vi "RT_Angular Aceleration in DLR Navigation Reference System(SubVI).vi"(0 "Mco (Nm)":dbl[](array[numeric]), 1 "MFE (Nm)":dbl[](array[numeric]), 2 "MFA (Nm)":dbl[](array[numeric]), 4 "MA_f [Nm]":dbl[](array[numeric]), 5 "MAd [Nm]":dbl[](array[numeric]), 7 "Rotation":T1, 9 "Data":dbl[][](array[numeric]), 11 "i":i32) -> (14 "ang_acc":dbl[](array[numeric]), 18 "ax/ay":dbl[](array[numeric]), 19 "Max/May":dbl[](array[numeric]))   [LabVIEW 2017]
uses:
  <vilib>/Analysis/_algsub.llb/Real PseudoInverse Matrix.vi
  <vilib>/Analysis/baseanly.llb/Real A x B.vi
  <vilib>/Analysis/Matrix/Numeric/Conversions/Array To Matrix - RA.vi
  <vilib>/Analysis/Matrix/Numeric/Conversions/Array To Matrix - RA2.vi
  <vilib>/Analysis/Matrix/Numeric/Conversions/Matrix To Array - RM.vi
  <vilib>/Analysis/NI_AALBase.lvlib
  <vilib>/Analysis/Matrix/NI_Matrix.lvlib
  <vilib>/Analysis/NI_AALPro.lvlib
panel:
  out "May":dbl
  out "Max":dbl
  out "ay":dbl
  out "ax":dbl
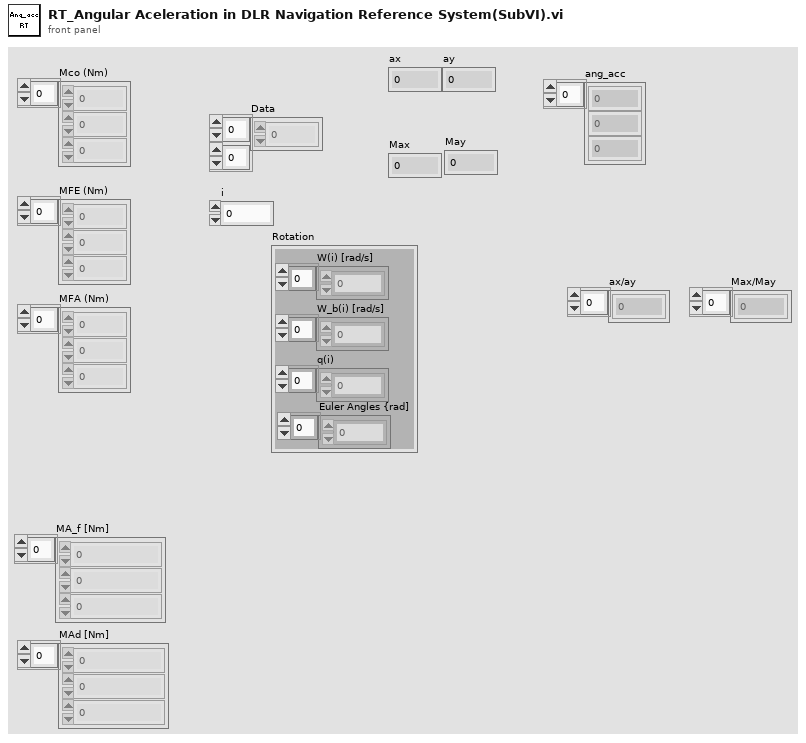
[diagram p1: front panel]
types:
  T1 = cluster{"W(i) [rad/s]":dbl[], "W_b(i) [rad/s]":dbl[], "q(i)":dbl[], "Euler Angles {rad]":dbl[]}
  T2 = typedef "NI_Matrix.lvlib/RealMatrix.ctl" = dbl[][]
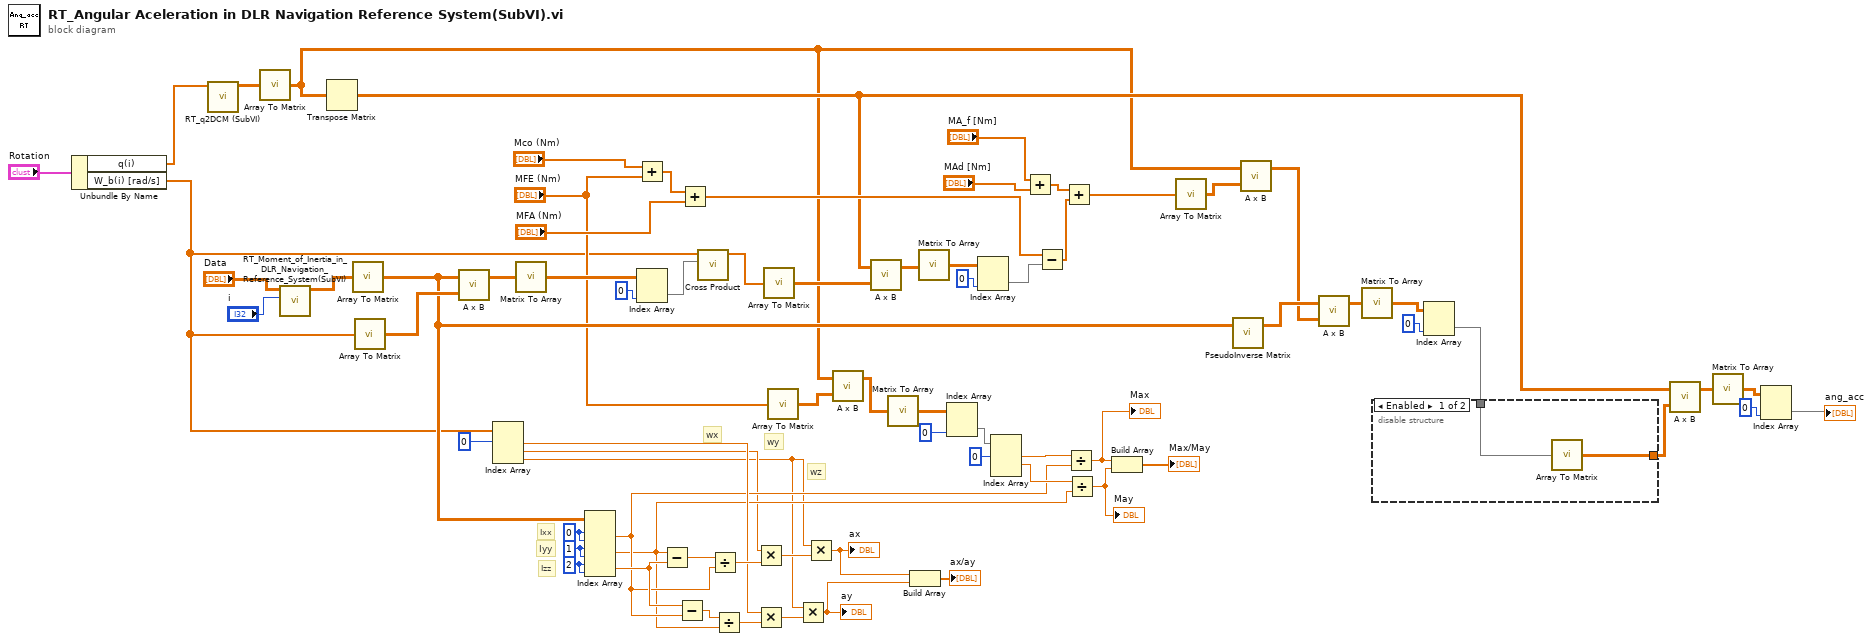
[diagram p0: block diagram]
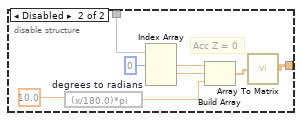
[diagram p2: hidden frame]
diagram:
  w34 = 2 ("index (row)")
  w35 = 1 ("index (row)")
  w36 = 0 ("index (row)")
  # "wz"
  # "wy"
  # "wx"
  # "Izz"
  # "Iyy"
  # "Ixx"
  n1 = Unbundle By Name("Rotation") -> ("q(i)"=w4:dbl[], "W_b(i) [rad/s]"=w3:dbl[])
  n2 = call "RT_q2DCM (SubVI).vi"("Quaternion"=w4) -> ("DCM"=w2:dbl[][])  [unwired: 10 in]
  n3 = call-poly <vilib>:"Array To Matrix.vi"("Real 2D Array"=w2) -> ("Real Matrix"=w19:T2)
  n4 = call "RT_Moment_of_Inertia_in_DLR_Navigation_Reference_System(SubVI).vi"("i"="i", "Data"="Data") -> ("I (kg.m^2)"=w58:dbl[][])  [unwired: 9 in]
  n5 = Transpose Matrix(1:w19) -> (0:w48:T2)
  n6 = call-poly <vilib>:"Array To Matrix.vi"("Real 2D Array"=w58) -> ("Real Matrix"=w37:T2)
  n7 = call-poly <vilib>:"Array To Matrix.vi"("Real 1D Array"=w3) -> ("Real Matrix (Column Vector)"=w69:T2)
  n8 = call-poly <vilib>:"A x B.vi"("B"=w69, "A"=w37) -> ("A x B"=w67:T2)  [unwired: 1 out]
  n9 = Index Array(array=w3, index #1=0 ("index (row)")) -> (element #1=w27:dbl, element #2=w6:dbl, element #3=w5:dbl)  [unwired: 2 in]
  n10 = call-poly <vilib>:"Matrix To Array.vi"("Real Matrix"=w67) -> ("Real 2D Array"=w68:dbl[][])
  n11 = Index Array(array=w37, index (row) #1=w36, index (col) #1=w36, index (row) #2=w35, index (col) #2=w35, index (row) #3=w34, index (col) #3=w34) -> (element #1=w10:dbl, element #2=w9:dbl, element #3=w31:dbl)
  n12 = Add(x="Mco (Nm)", y="MFE (Nm)") -> (x+y=w63:dbl[])
  n13 = Index Array(array=w68, index (col)=0 ("index (row)")) -> (element=w70:dbl[])  [unwired: 1 in]
  n14 = Subtract(x=w9, y=w31) -> (x-y=w32:dbl)
  n15 = Subtract(x=w31, y=w10) -> (x-y=w30:dbl)
  n16 = Add(x=w63, y="MFA (Nm)") -> (x+y=w64:dbl[])
  n17 = call <vilib>:"Cross Product.vi"("B Vector"=w70, "A Vector"=w3) -> ("Cross Product"=w57:dbl[])  [unwired: 8 in, 1 out]
  n18 = Divide(x=w32, y=w10) -> (x/y=w29:dbl)
  n19 = Divide(x=w30, y=w9) -> (x/y=w28:dbl)
  n20 = Multiply(x=w6, y=w29) -> (x*y=w26:dbl)
  n21 = Multiply(x=w27, y=w28) -> (x*y=w25:dbl)
  n22 = call-poly <vilib>:"Array To Matrix.vi"("Real 1D Array"=w57) -> ("Real Matrix (Column Vector)"=w56:T2)
  n23 = call-poly <vilib>:"Array To Matrix.vi"("Real 1D Array"="MFE (Nm)") -> ("Real Matrix (Column Vector)"=w21:T2)
  n24 = Multiply(x=w5, y=w25) -> (x*y=w23:dbl)
  "ay" <- w23
  n25 = Multiply(x=w5, y=w26) -> (x*y=w24:dbl)
  "ax" <- w24
  n26 = call-poly <vilib>:"A x B.vi"("B"=w21, "A"=w19) -> ("A x B"=w16:T2)  [unwired: 1 out]
  n27 = call-poly <vilib>:"A x B.vi"("B"=w56, "A"=w48) -> ("A x B"=w53:T2)  [unwired: 1 out]
  n28 = call-poly <vilib>:"Matrix To Array.vi"("Real Matrix"=w16) -> ("Real 2D Array"=w17:dbl[][])
  n29 = Build Array(w24, w23) -> (→"ax/ay":dbl[])
  n30 = call-poly <vilib>:"Matrix To Array.vi"("Real Matrix"=w53) -> ("Real 2D Array"=w54:dbl[][])
  n31 = Index Array(array=w17, index (col)=0 ("index (row)")) -> (element=w15:dbl[])  [unwired: 1 in]
  n32 = Index Array(array=w54, index (col)=0 ("index (row)")) -> (element=w52:dbl[])  [unwired: 1 in]
  n33 = Index Array(array=w15, index #1=0 ("index (row)")) -> (element #1=w12:dbl, element #2=w11:dbl)  [unwired: 2 in, 1 out]
  n34 = Add(x="MA_f [Nm]", y="MAd [Nm]") -> (x+y=w41:dbl[])
  n35 = Subtract(x=w64, y=w52) -> (x-y=w42:dbl[])
  n36 = Add(x=w41, y=w42) -> (x+y=w43:dbl[])
  n37 = Divide(x=w12, y=w10) -> (x/y=w7:dbl)
  "Max" <- w7
  n38 = Divide(x=w11, y=w9) -> (x/y=w8:dbl)
  "May" <- w8
  n39 = Build Array(w7, w8) -> (→"Max/May":dbl[])
  n40 = call-poly <vilib>:"Array To Matrix.vi"("Real 1D Array"=w43) -> ("Real Matrix (Column Vector)"=w51:T2)
  n41 = call-poly <vilib>:"PseudoInverse Matrix.vi"("Input Matrix"=w37) -> ("PseudoInverse Matrix"=w71:T2)  [unwired: 1 in, 1 out]
  n42 = call-poly <vilib>:"A x B.vi"("B"=w51, "A"=w19) -> ("A x B"=w50:T2)  [unwired: 1 out]
  n43 = call-poly <vilib>:"A x B.vi"("B"=w50, "A"=w71) -> ("A x B"=w72:T2)  [unwired: 1 out]
  n44 = call-poly <vilib>:"Matrix To Array.vi"("Real Matrix"=w72) -> ("Real 2D Array"=w73:dbl[][])
  n45 = Index Array(array=w73, index (col)=0 ("index (row)")) -> (element=w38:dbl[])  [unwired: 1 in]
  n46 = disable-structure shown="Enabled" {
    disable-tunnel: [w75 w78] -> w47
    disable-tunnel: w38 -> [w74 w82]
    frame Enabled {
      n47 = call-poly <vilib>:"Array To Matrix.vi"("Real 1D Array"=w74) -> ("Real Matrix (Column Vector)"=w75:T2)
    }
    frame Disabled {
      # "Acc Z = 0"
      n48 = expression code="(x/180.0)*pi" "degrees to radians"(10.0 ("element")) -> (w76:dbl)
      n49 = Index Array(array=w82, index #1=0 ("index")) -> (element #1=w81:dbl, element #2=w80:dbl)  [unwired: 2 in, 1 out]
      n50 = Build Array(w81, w80, w76) -> (w79:dbl[])
      n51 = call-poly <vilib>:"Array To Matrix.vi"("Real 1D Array"=w79) -> ("Real Matrix (Column Vector)"=w78:T2)
    }
  }
  n52 = call-poly <vilib>:"A x B.vi"("B"=w47, "A"=w48) -> ("A x B"=w49:T2)  [unwired: 1 out]
  n53 = call-poly <vilib>:"Matrix To Array.vi"("Real Matrix"=w49) -> ("Real 2D Array"=w45:dbl[][])
  n54 = Index Array(array=w45, index (col)=0 ("index (row)")) -> (element=→"ang_acc":dbl[])  [unwired: 1 in]
